vi "F Dwf Digital I2c Write.vi"(6 "pNak":i32, 7 "cTx":i32, 8 "error in (no error)":errorcluster, 9 "rgbTx":string, 10 "adr8bits":u8, 11 "hdwf":i32) -> (0 "error out":errorcluster, 1 "rgbTx out":string, 3 "function return":i32, 4 "pNak out":i32)   [LabVIEW 2019, in "Olasdwf.lvlib"]
doc: "DWFAPI int FDwfDigitalI2cWrite(HDWF hdwf, unsigned char adr8bits, unsigned char *rgbTx, int cTx, int *pNak);"
uses:
  Olasdwf.lvlib
  Windows/System32/dwf.dll
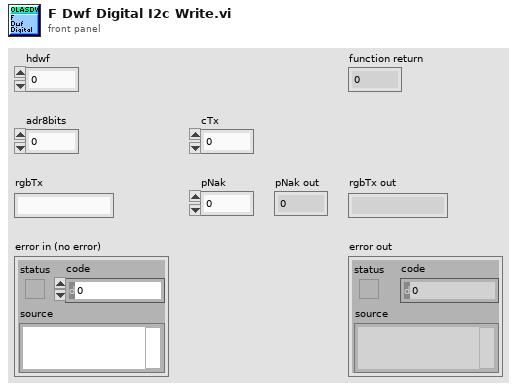
[diagram p1: front panel]
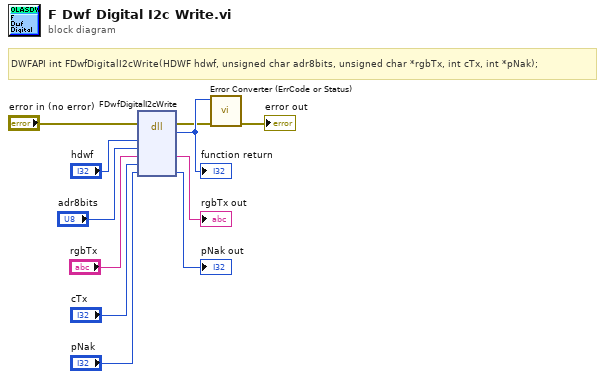
[diagram p0: block diagram]
diagram:
  # "DWFAPI int FDwfDigitalI2cWrite(HDWF hdwf, unsigned char adr8bits, unsigned char *rgbTx, int cTx, int *pNak);"
  n1 = dll-call lib="C:/Windows/System32/dwf.*" fn="FDwfDigitalI2cWrite"(error in="error in (no error)", "hdwf"="hdwf", "adr8bits"="adr8bits", "rgbTx"="rgbTx", "cTx"="cTx", "pNak"="pNak") -> (error out=w2:errorcluster, w11:i32, "rgbTx"=→"rgbTx out":string, "pNak"=→"pNak out":i32)  [unwired: 5 in, 1 out]
  "function return" <- w11
  n2 = call "Error Converter (ErrCode or Status).vi"("error in (no error)"=w2, "error code"=w11) -> ("error out"=→"error out":errorcluster)  [unwired: 9 in]
